vi "Write Draw Component.vi"(8 "error in (no error)":errorcluster, 10 "DrawComponent.lvclass":refnum<class "DrawComponent.lvclass">, 11 "SimulationObject in":refnum<class "SimulationObject.lvclass">) -> (0 "error out":errorcluster, 3 "SimulationObject out":refnum<class "SimulationObject.lvclass">)   [LabVIEW 2022 SP3, in "SimulationObject.lvclass"]
uses:
  SimulationObject.lvclass
  SimulationObject.lvclass/SimulationObject.ctl
  Components/DrawComponent/DrawComponent.lvclass
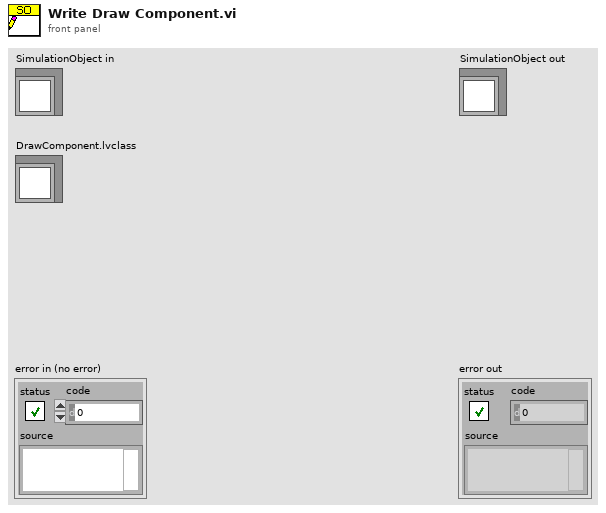
[diagram p1: front panel]
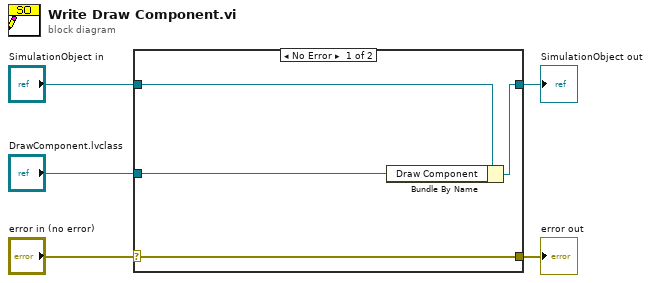
[diagram p0: block diagram]
diagram:
  n1 = case shown="No Error" "error in (no error)" {
    selector: "error in (no error)" -> [w9 w10]
    tunnel: [w9 w10] -> w4
    tunnel: [w7 w11] -> w2
    tunnel: "SimulationObject in" -> [w8 w11]
    tunnel: "DrawComponent.lvclass" -> [w6 _]
    frame No Error {
      n2 = Bundle By Name(cluster=w8, "Draw Component"=w6) -> (w7:refnum<class "SimulationObject.lvclass">)
    }
    frame Error {
    }
  }
  "error out" <- w4
  "SimulationObject out" <- w2
